vi "CODMn启动命令 (子VI).vi"(9 "强制切换":bool, 10 "CODMn量程切换":enum32{"H", "L", "AUTO"}(ring)=enum."AUTO", 11 "启动测量模式":T1) -> ()   [LabVIEW 2016, in "斯坦道CODMn.lvlib"]
uses:
  <vilib>/Plasmionique/MB Master/MB_Master_Serial/MB_Master_Serial.lvclass
  D:/Program Files (x86)/National Instruments/LabVIEW 2016/vi.lib/Plasmionique/MB Master/MB_Master/MB_Master.lvclass
  <vilib>/Plasmionique/MB Master/MB Master.lvlib
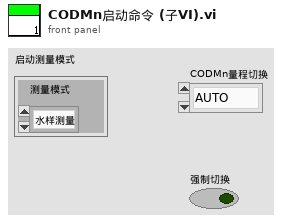
[diagram p1: front panel]
types:
  T1 = cluster{"测量模式":enum16{"水样测量", "标样核查", "零点核查", "跨度核查", "空白测试", "加标回收", "平行样", "校零", "校标"}}
  T2 = cluster{"baud rate (bps)":u32, "stop bits":u16, "parity":u16, "flow control":u16, "timeout":u32, "retries":i32}
  T3 = enum16{"水样测量", "标样核查", "零点核查", "跨度核查", "空白测试", "加标回收", "平行样", "校零", "校标"}
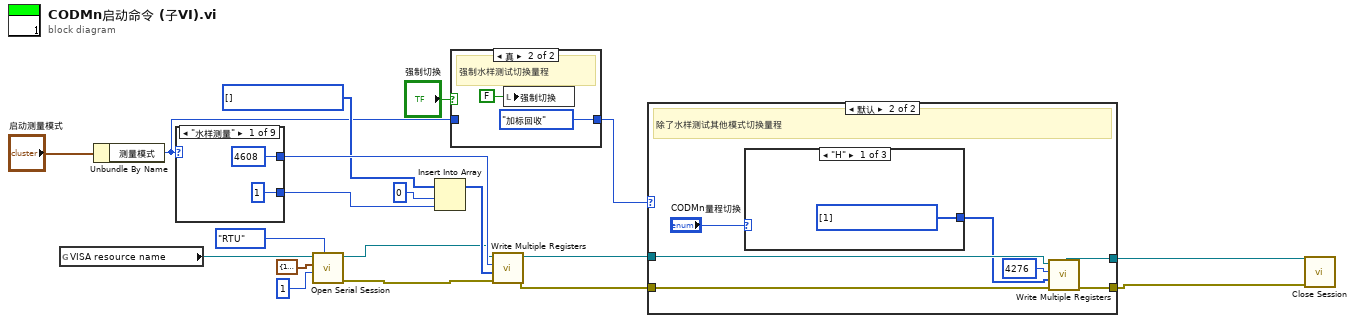
[diagram p0: block diagram]
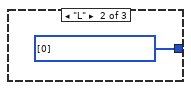
[diagram p4: hidden frame]
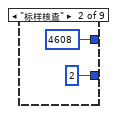
[diagram p6: hidden frame]
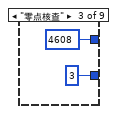
[diagram p7: hidden frame]
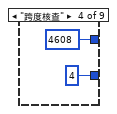
[diagram p8: hidden frame]
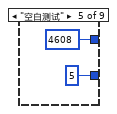
[diagram p9: hidden frame]
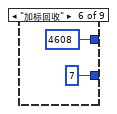
[diagram p10: hidden frame]
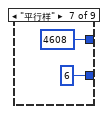
[diagram p11: hidden frame]
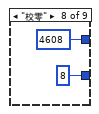
[diagram p12: hidden frame]
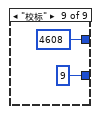
[diagram p13: hidden frame]
diagram:
  n1 = global read "COD浓度全局变量.vi" "VISA resource name"() -> (w6:refnum<visa-resource-name>)
  n2 = Unbundle By Name("启动测量模式") -> ("测量模式"=w3:T3)
  n3 = case shown="\"水样测量\"" w3 {
    tunnel: [u16 4608 ("address") u16 4608 ("address") u16 4608 ("address") u16 4608 ("address") u16 4608 ("address") u16 4608 ("address") u16 4608 ("address") u16 4608 ("address") u16 4608 ("address")] -> w18
    tunnel: [u16 1 ("address") u16 2 ("address") u16 3 ("address") u16 4 ("address") u16 5 ("address") u16 7 ("address") u16 6 ("address") u16 8 ("address") u16 9 ("address")] -> w13
    frame "水样测量" {
    }
    frame "标样核查" {
    }
    frame "零点核查" {
    }
    frame "跨度核查" {
    }
    frame "空白测试" {
    }
    frame "加标回收" {
    }
    frame "平行样" {
    }
    frame "校零" {
    }
    frame "校标" {
    }
  }
  n4 = call <vilib>:"Open Serial Session.vi"("Mode (RTU)"=enum16{"RTU", "ASCII"}."RTU", "Slave ID"=u8 1, "Serial Config"=T2 {"baud rate (bps)"=115200, "stop bits"=10, "parity"=0, "flow control"=0, "timeout"=1000, "retries"=1}, "VISA Resource"=w6) -> ("Error out"=w4:errorcluster, "MB_Serial session"=w5:refnum<class "MB_Master_Serial.lvclass">)  [unwired: 6 in]
  n5 = Insert Into Array(array=u16[] [] ("values"), index=0 ("索引"), new element=w13) -> (w19:u16[])
  n6 = case shown="真" "强制切换" {
    tunnel: w3 -> [w38 _]
    tunnel: [w38 T3."加标回收" ("测量模式")] -> w2
    frame False {
    }
    frame True {
      # "强制水样测试切换量程"
      n7 = local write "强制切换"(FALSE ("强制切换")) -> ()
    }
  }
  n8 = call <vilib>:"Write Multiple Registers.vi"("error in (no error)"=w4, "values"=w19, "starting address"=w18, "MB session in"=w5) -> ("error out"=w9:errorcluster, "MB session out"=w10:refnum<class "MB_Master_Serial.lvclass">)  [unwired: 6 in]
  n9 = case shown="默认" w2 {
    tunnel: w10 -> [w42 w49]
    tunnel: w9 -> [w41 w48]
    tunnel: [w42 w47] -> w8
    tunnel: [w41 w46] -> w7
    frame "水样测量" {
      # "水样测试不切换"
    }
    frame Default {
      # "除了水样测试其他模式切换量程"
      n10 = case shown="\"H\"" "CODMn量程切换" {
        tunnel: [u16[] [1] ("values") u16[] [0] ("values") _] -> w43
        frame "H" {
        }
        frame "L" {
        }
        frame "AUTO", Default {
        }
      }
      n11 = call <vilib>:"Write Multiple Registers.vi"("error in (no error)"=w48, "values"=w43, "starting address"=u16 4276, "MB session in"=w49) -> ("error out"=w46:errorcluster, "MB session out"=w47:refnum<class "MB_Master_Serial.lvclass">)  [unwired: 6 in]
    }
  }
  n12 = call-dynamic "Close Session.vi"("error in (no error)"=w7, "MB_Serial session"=w8) -> ()  [unwired: 9 in, 1 out]
